vi "Get State.vi"(8 "error in (no error)":errorcluster, 11 "DAQmx Digitizer in":refnum<class "DAQmx Synthesizer.lvclass">) -> (0 "error out":errorcluster, 1 "Data ready":bool, 2 "Armed":bool, 3 "DAQmx Digitizer out":refnum<class "DAQmx Synthesizer.lvclass">, 4 "Availiable Samples":u32, 5 "Finished":bool)   [LabVIEW 2019, in "DAQmx Synthesizer.lvclass"]
uses:
  DAQmx Synthesizer.lvclass
  DAQmx Synthesizer.lvclass/DAQmx Synthesizer.ctl
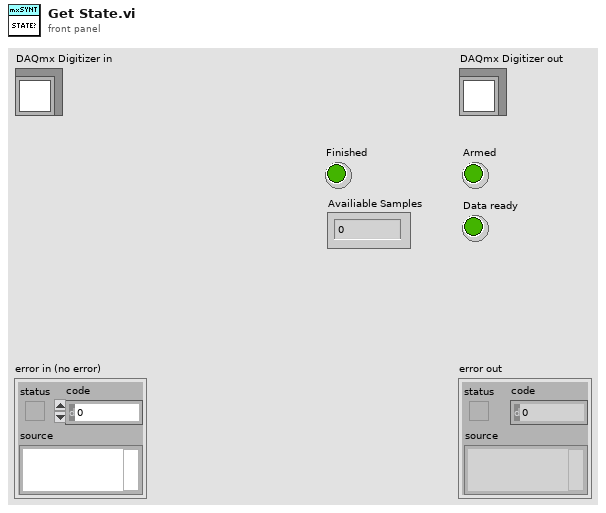
[diagram p1: front panel]
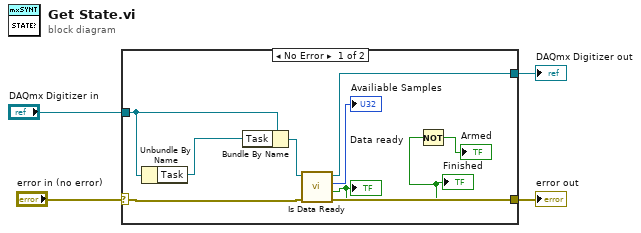
[diagram p0: block diagram]
diagram:
  n1 = case shown="No Error" "error in (no error)" {
    selector: "error in (no error)" -> [w12 w15]
    tunnel: [w6 w15] -> w3
    tunnel: [w9 w14] -> w1
    tunnel: "DAQmx Digitizer in" -> [w13 w14]
    frame No Error {
      n2 = Unbundle By Name(w13) -> ("Task"=w11:refnum<k21>)
      n3 = Bundle By Name(cluster=w13, "Task"=w11) -> (w8:refnum<class "DAQmx Synthesizer.lvclass">)
      n4 = call-dynamic "Is Data Ready.vi"("error in (no error)"=w12, "DAQmx Digitizer in"=w8) -> ("error out"=w6:errorcluster, "Data ready"=w5:bool, "Availiable Samples"=→"Availiable Samples":u32, "DAQmx Digitizer out"=w9:refnum<class "DAQmx Synthesizer.lvclass">)  [unwired: 6 in]
      "Finished" <- w5
      "Data ready" <- w5
      n5 = Not(x=w5) -> (.not. x?=→"Armed":bool)
    }
    frame Error {
    }
  }
  "error out" <- w3
  "DAQmx Digitizer out" <- w1
